vi "Async VI Control_Clear Trigger.vi"(6 "Parent VI":refnum<vi>, 8 "error in (no error)":errorcluster) -> (0 "error out":errorcluster)   [LabVIEW 2021, in "CANOpen Addon Engine.lvlib"]
uses:
  CANOpen Addon Engine.lvlib
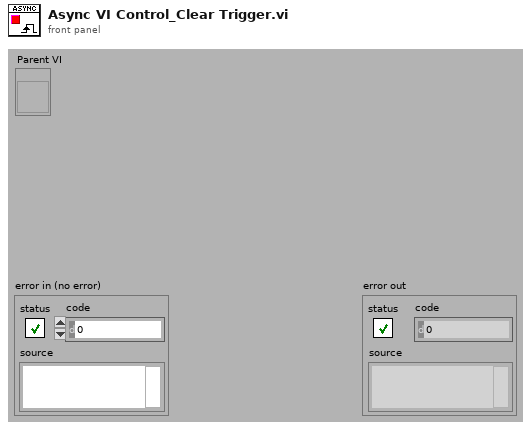
[diagram p1: front panel]
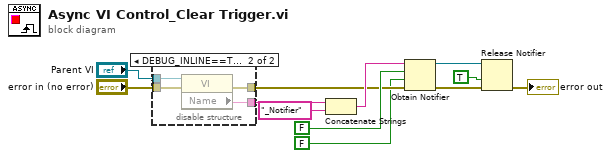
[diagram p0: block diagram]
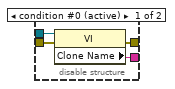
[diagram p2: hidden frame]
diagram:
  n1 = disable-structure shown="DEBUG_INLINE==TRUE" {
    disable-tunnel: [w16 w20] -> w10
    disable-tunnel: [w15 w19] -> w6
    disable-tunnel: "error in (no error)" -> [w14 w18]
    disable-tunnel: "Parent VI" -> [w13 w17]
    frame condition #0 (active) {
      n2 = property class="VI"(reference=w13, error in=w14) -> (error out=w15:errorcluster, "Clone Name"=w16:string)  [unwired: 1 out]
    }
    frame condition #1 {
      n3 = property class="VI"(reference=w17, error in=w18) -> (error out=w19:errorcluster, "Name"=w20:string)  [unwired: 1 out]
    }
  }
  n4 = Concatenate Strings(w10, "_Notifier" ("name (unnamed)")) -> (w8:string)
  n5 = Obtain Notifier(name (unnamed)=w8, notification data type=FALSE, create if not found? (T)=FALSE, error in (no error)=w6) -> (notifier out=w1:refnum<notifier>, error out=w3:errorcluster)  [unwired: 1 out]
  n6 = Release Notifier(notifier=w1, force destroy? (F)=TRUE ("notification"), error in (no error)=w3) -> (error out=→"error out":errorcluster)  [unwired: 2 out]
